vi "DQtoAlphaBeta_noSine_src.vi"(0 "direct":sgl format="%#_30g", 1 "cosx":sgl, 2 "sinx":sgl, 5 "quadrature":sgl format="%#_30g") -> (4 "alpha":sgl format="%#_30g", 6 "beta":sgl format="%#_30g")   [LabVIEW 2015]
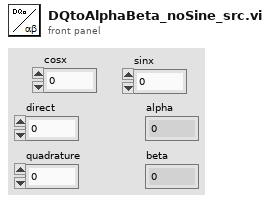
[diagram p1: front panel]
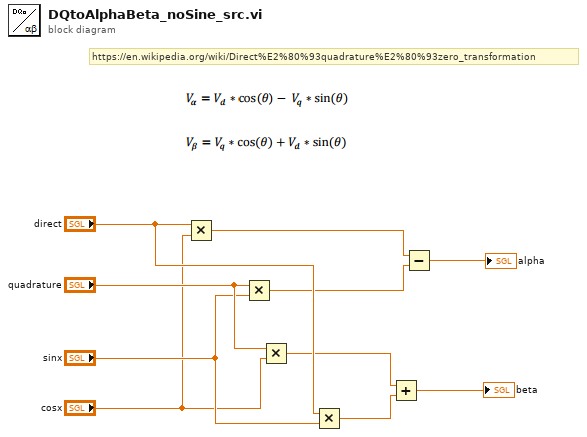
[diagram p0: block diagram]
diagram:
  # "https://en.wikipedia.org/wiki/Direct%E2%80%93quadrature%E2%80%93zero_transformation"
  n1 = Multiply(x="direct", y="cosx") -> (x*y=w6:sgl)
  n2 = Multiply(x="quadrature", y="sinx") -> (x*y=w5:sgl)
  n3 = Multiply(x="quadrature", y="cosx") -> (x*y=w8:sgl)
  n4 = Multiply(x="direct", y="sinx") -> (x*y=w7:sgl)
  n5 = Add(x=w8, y=w7) -> (x+y=→"beta":sgl)
  n6 = Subtract(x=w6, y=w5) -> (x-y=→"alpha":sgl)
